vi "New D_Datagrid.vi"(6 "Scrolling mode (default)":T1, 8 "Owning VI (caller)":refnum<vi>, 9 "Auto update indicator? (T)":bool=TRUE, 10 "Indicator reference":refnum<vi>, 11 "D_Datagrid in":refnum<class "D_Datagrid.lvclass">) -> (0 "error out":errorcluster, 1 "Programmatic edit launch":refnum<user-event>, 2 "Element touched event":refnum<user-event>, 3 "D_Datagrid out":refnum<class "D_Datagrid.lvclass">)   [LabVIEW 2023, in "D Datagrid Library.lvlib" / "D_Datagrid.lvclass"]
doc: "This VI creates the background information for the D_Datagrid control. It supplies the Element Touched event refnum, which fires when a user \"touches\" an Enabled element. It includes NewVal, OldVal, and a Changed? boolean. A Touch can be simply clicking the value and opening the field, then typing the same value, or pressing Escape. The <Owning VI> is an optional input to fix bugs relating to subpanels. If the VI is going in a subpanel, wire the topmost VI reference to this terminal."
uses:
  D_Datagrid.lvclass
  D_Datagrid.lvclass/D_Datagrid.ctl
  DatagridElement/DatagridElement.lvclass
  D Datagrid Update Element.ctl
  <vilib>/Utility/miscctls.llb/LVRowAndColumnTypeDef.ctl
  Scrolling behavior.ctl
panel:
  # "Generates a user event on value change,\nincluding the row, column, and new element."
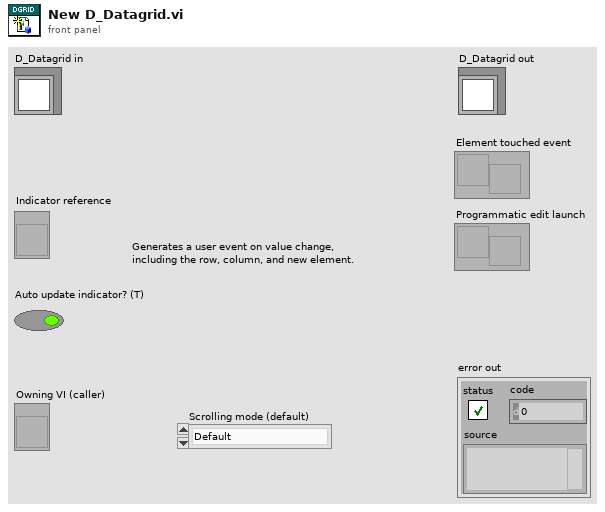
[diagram p1: front panel]
types:
  T1 = typedef "D Datagrid Library.lvlib/D_Datagrid.lvclass/Scrolling behavior.ctl" = enum16{"Default", "Locked", "Displayed items only"}
  T2 = typedef "LVRowAndColumnTypeDef.ctl" = cluster{"Row":i32, "Column":i32}
  T3 = typedef "D Datagrid Library.lvlib/D_Datagrid.lvclass/D Datagrid Update Element.ctl" = cluster{"Row":i32, "Column":i32, "Element NewVal":refnum<class "DatagridElement.lvclass">, "Element OldVal":refnum<class "DatagridElement.lvclass">, "Changed?":bool}
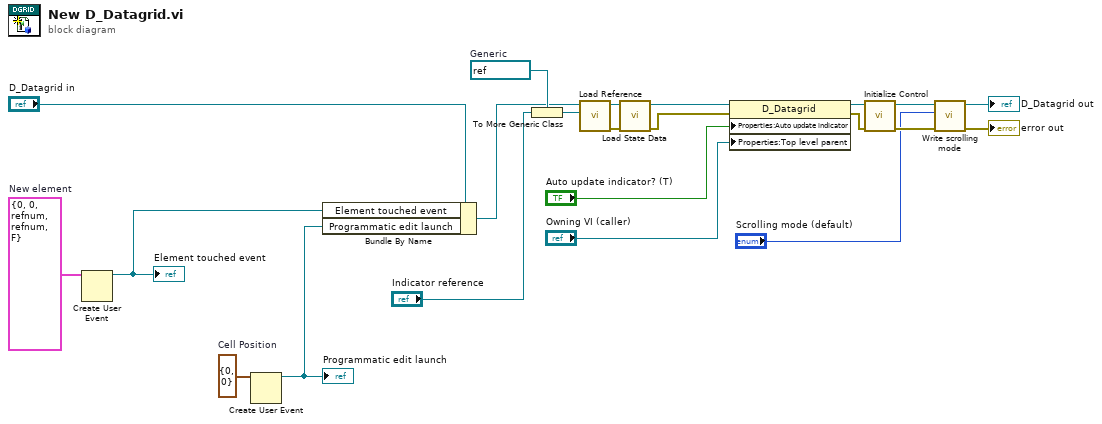
[diagram p0: block diagram]
diagram:
  w13 = T2 {"Row"=0, "Column"=0}  # Cell Position
  w18 = T3 {"Row"=0, "Column"=0, "Element NewVal"=refnum, "Element OldVal"=refnum, "Changed?"=FALSE}  # New element
  w21 = refnum<vi> refnum  # Generic
  n1 = Create User Event(user event datatype=w18) -> (user event=w17:refnum<user-event>)  [unwired: 1 in, 1 out]
  "Element touched event" <- w17
  n2 = Create User Event(user event datatype=w13) -> (user event=w12:refnum<user-event>)  [unwired: 1 in, 1 out]
  "Programmatic edit launch" <- w12
  n3 = Bundle By Name(cluster="D_Datagrid in", "Element touched event"=w17, "Programmatic edit launch"=w12) -> (w16:refnum<class "D_Datagrid.lvclass">)
  n4 = To More Generic Class(target class=w21, reference="Indicator reference") -> (generic class reference=w22:refnum<vi>)
  n5 = call-dynamic "Load Reference.vi"("Reference"=w22, "D_Datagrid in"=w16) -> ("error out"=w20:errorcluster, "D_Datagrid out"=w19:refnum<class "D_Datagrid.lvclass">)  [unwired: 8 in]
  n6 = call-dynamic "Load State Data.vi"("error in (no error)"=w20, "D_Datagrid in"=w19) -> ("error out"=w7:errorcluster, "D_Datagrid out"=w8:refnum<class "D_Datagrid.lvclass">)  [unwired: 8 in]
  n7 = property class="D_Datagrid"(reference=w8, error in=w7, "Properties:Auto update indicator"="Auto update indicator? (T)", "Properties:Top level parent"="Owning VI (caller)") -> (reference out=w10:refnum<class "D_Datagrid.lvclass">, error out=w9:errorcluster)
  n8 = call-dynamic "Initialize Control.vi"("error in (no error)"=w9, "D_Datagrid in"=w10) -> ("error out"=w5:errorcluster, "D_Datagrid out"=w4:refnum<class "D_Datagrid.lvclass">)  [unwired: 8 in]
  n9 = call "Write scrolling mode.vi"("error in (no error)"=w5, "Scrolling mode"="Scrolling mode (default)", "D_Datagrid in"=w4) -> ("error out"=→"error out":errorcluster, "D_Datagrid out"=→"D_Datagrid out":refnum<class "D_Datagrid.lvclass">)  [unwired: 7 in]
